vi "Main_FFT.vi"() -> ()   [LabVIEW 2026]
doc: "This template is for the Queued Message Handler design pattern.\n\nThe Event Handling Loop generates messages based on user interface actions.\n\nThe Message Handling Loop processes messages generated by the Event Handling Loop, or by other messages. The messages are string values, so new messages can be added easily to the Message Cases case structure in the Message Handling Loop. Each message cluster can also provide an optional value for Message Data, which is a variant that can be converted to whatever message-specific data is required."
uses:
  SubVIs/Controls/PCO_Config.ctl
  SubVIs/Controls/UI Data.ctl
  SubVIs/pco.labview/camera/Camera.lvclass
  SubVIs/Controls/TypeDef_FGV.ctl
  SubVIs/QMH/Message Queue/Enqueue Message (Single).vi
  SubVIs/QMH/Message Queue/Message Queue.lvlib
  SubVIs/QMH/User Event - Stop/User Event - Stop.lvlib
  SubVIs/pco.labview/pco.sdk/TimingControl/TimingControl.lvlib
panel:
  in  "# of frames":u16=100
  in  "SavePath":path=path "E:/exp_data/Seb"
  out "FFT":dbl[][](graph)
  out "Graphe d'intensité":u16[][](graph)
  in  "Binning for FFT":u16(ring)=8 items=["1x1"=1, "2x2"=2, "4x4"=4, "8x8"=8]
  in  "Stop live":bool
  in  "FFT?":bool=TRUE
  in  "Grab":bool
  in  "Live":bool
  in  "PCO_Config":T1={"Exposure time (s)"=0.01, "TriggerMode"=0, "ROI X0"=1, "ROI Y0"=1, "ROI X1"=2048, "ROI Y1"=2048, "Binning"=1} {"TriggerMode" items=["auto sequence", "software trigger", "external exposure start", "external exposure control"]}
  out "Current task":string="\"Exit\" button pressed"
  in  "Exit":bool
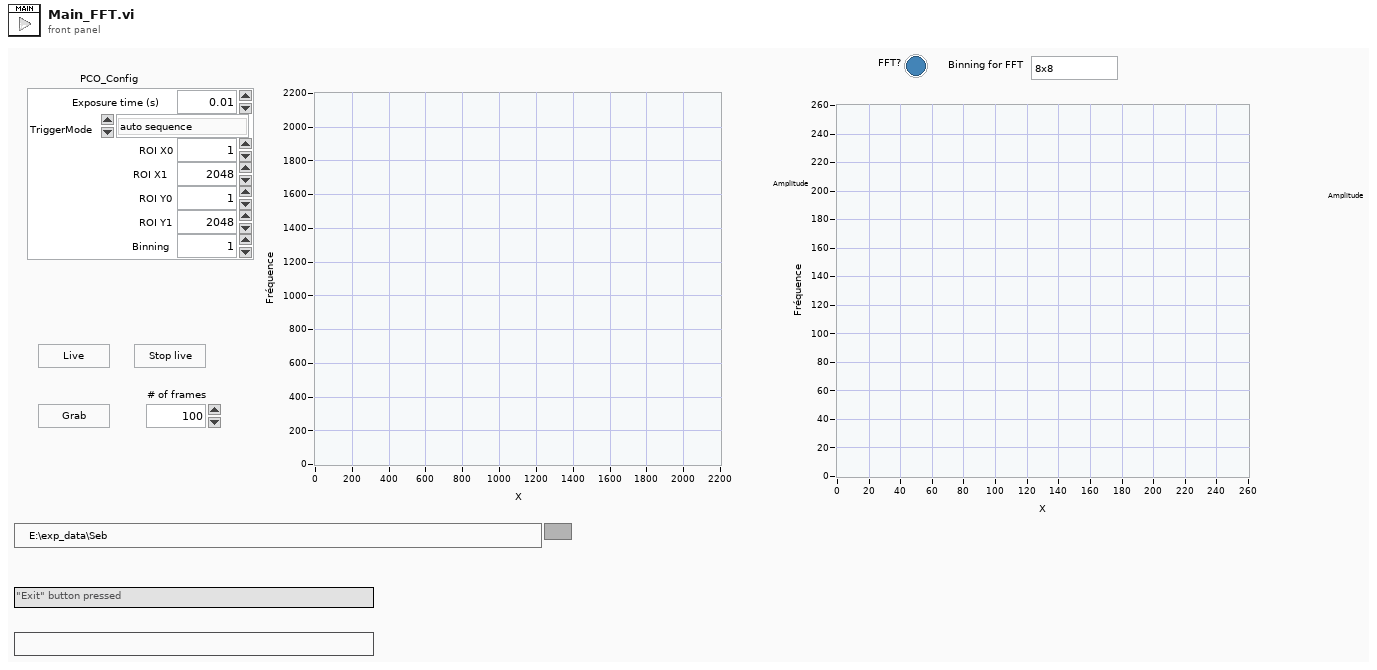
[diagram p1: front panel]
types:
  T1 = typedef "PCO_Config.ctl" = cluster{"Exposure time (s)":dbl, "TriggerMode":u16, "ROI X0":u16, "ROI Y0":u16, "ROI X1":u16, "ROI Y1":u16, "Binning":u8}
  T2 = typedef "UI Data.ctl" = cluster{"Data Display Ref":refnum<vi>, "Exit Button Ref":refnum<vi>, "Message":string}
  T3 = typedef "Message Queue.lvlib/All Message Queues.ctl" = cluster{"UI":refnum<queue>, "Camera loop":refnum<queue>, "Display loop":refnum<queue>}
  T4 = typedef "TypeDef_FGV.ctl" = enum16{"Initialize", "Write", "Read"}
  T5 = enum16{"auto sequence", "software trigger", "external exposure start", "external exposure control"}
  T6 = typedef "Camera.lvclass/binning.ctl" = cluster{"vert":u16, "horz":u16, "mode":u16}
  T7 = cluster{"exposure_time_s":dbl, "delay_time_s":dbl, "roi":cluster{"x0":u64, "y0":u64, "x1":u64, "y1":u64}, "timestamp_mode":u16, "pixelrate":u32, "conversion_factor":sgl, "trigger_mode":u16, "acquire_mode":u16, "acquire_sequence_number":u32, "metadata_mode":u16, "noisefilter_mode":u16, "pixel_format":u32, "binning":T6, "auto_exposure":cluster{"region":u16, "min_exposure_s":dbl, "max_exposure_s":dbl}}
  T8 = cluster{"wSignalNum":u16, "wEnabled":u16, "wType":u16, "wPolarity":u16, "wFilterSetting":u16, "wSelected":u16, "dwParameter":u32[], "dwSignalFunctionality":u32[]}
  T9 = cluster{"wVersion":u16, "dwIMAGE_COUNTER":u32, "dwIMAGE_TIME_US":u32, "lvTimestamp":timestamp, "bIMAGE_TIME_STATUS":u8, "wEXPOSURE_TIME_BASE":u16, "dwEXPOSURE_TIME":u32, "dwFRAMERATE_MILLIHZ":u32, "sSENSOR_TEMPERATURE":i16, "wIMAGE_SIZE_X":u16, "wIMAGE_SIZE_Y":u16, "bBINNING_X":u8, "bBINNING_Y":u8, "dwSENSOR_READOUT_FREQUENCY":u32, "wSENSOR_CONV_FACTOR":u16, "dwCAMERA_SERIAL_NO":u32, "wCAMERA_TYPE":u16, "bBIT_RESOLUTION":u8, "bSYNC_STATUS":u8, "wDARK_OFFSET":u16, "bTRIGGER_MODE":u8, "bDOUBLE_IMAGE_MODE":u8, "bCAMERA_SYNC_MODE":u8, "bIMAGE_TYPE":u8, "wCOLOR_PATTERN":u16, "wCAMERA_SUBTYPE":u16, "dwEVENT_NUMBER":u32, "wIMAGE_SIZE_X_Offset":u16, "wIMAGE_SIZE_Y_Offset":u16, "bREADOUT_MODE":u8}[]
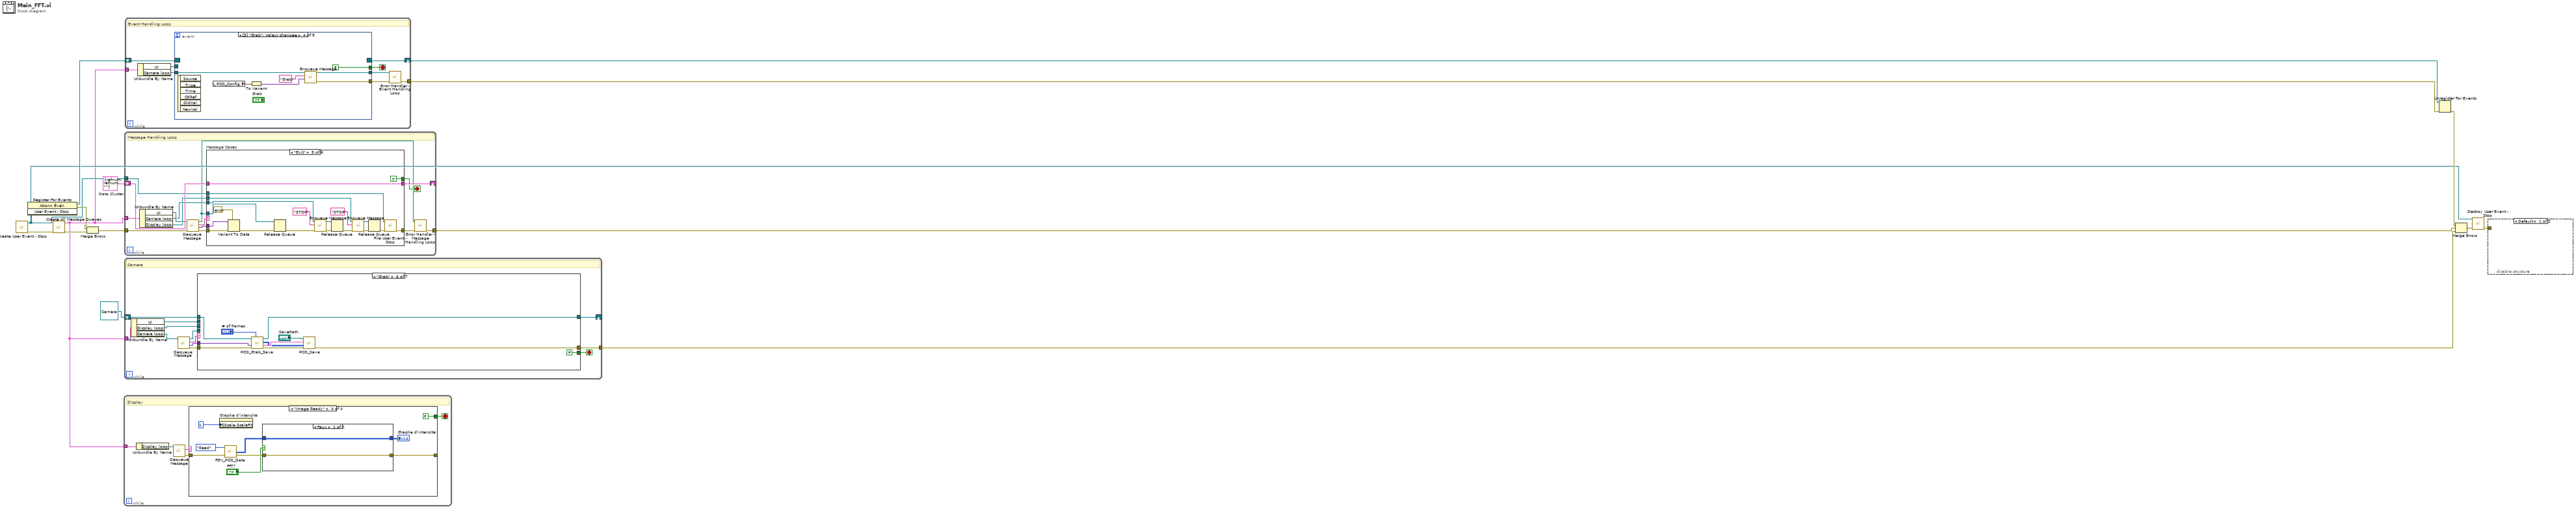
[diagram p0: block diagram]
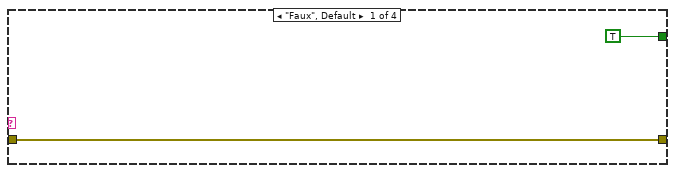
[diagram p2: hidden frame]
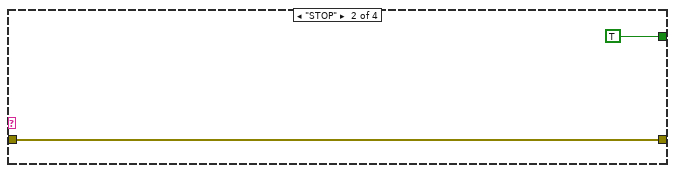
[diagram p3: hidden frame]
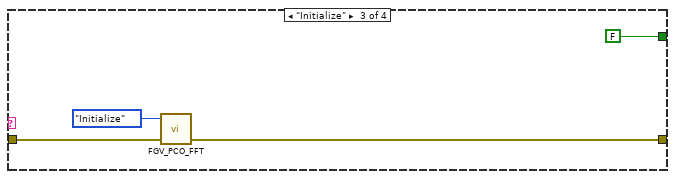
[diagram p4: hidden frame]
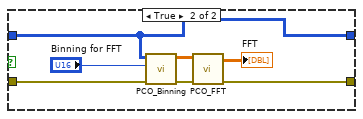
[diagram p5: hidden frame]
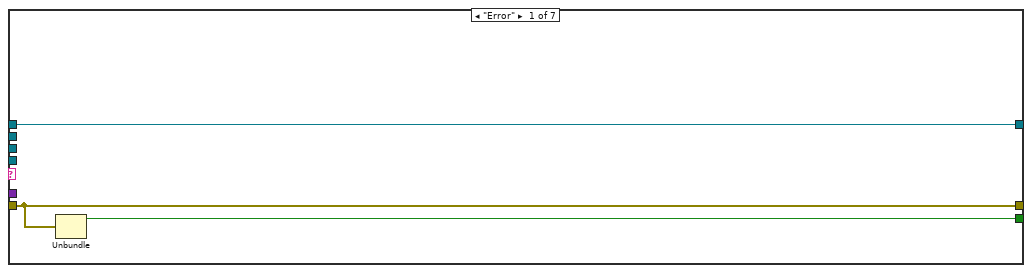
[diagram p6: hidden frame]
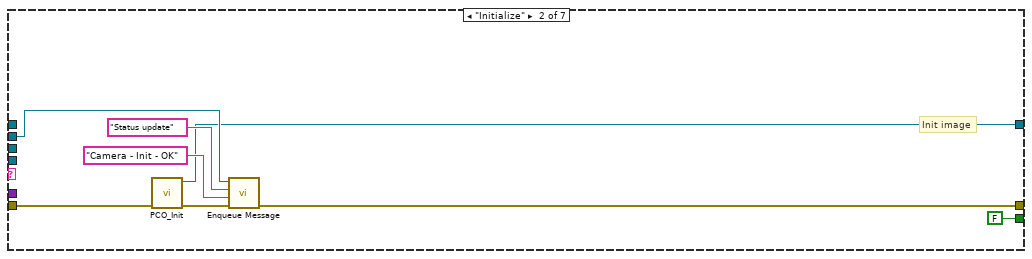
[diagram p7: hidden frame]
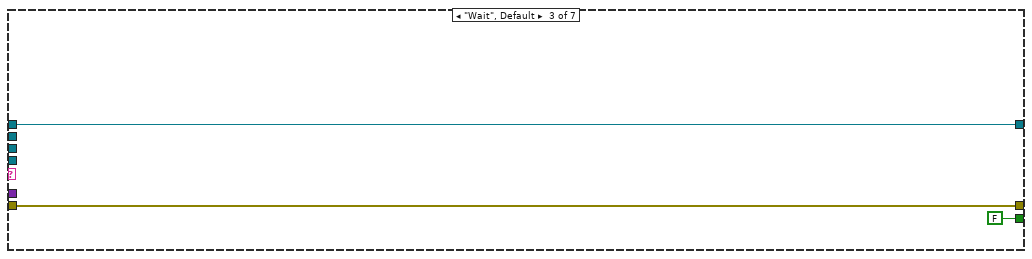
[diagram p8: hidden frame]
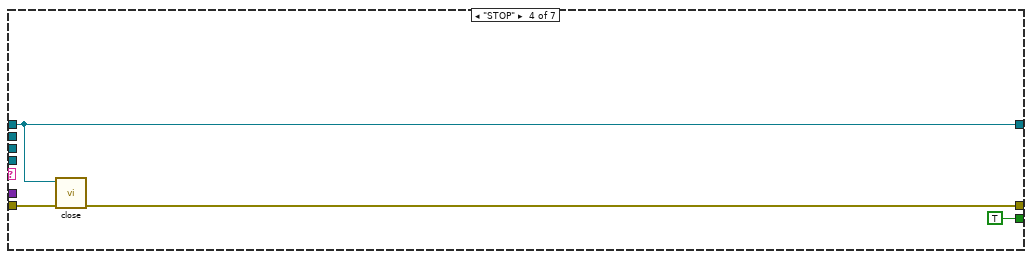
[diagram p9: hidden frame]
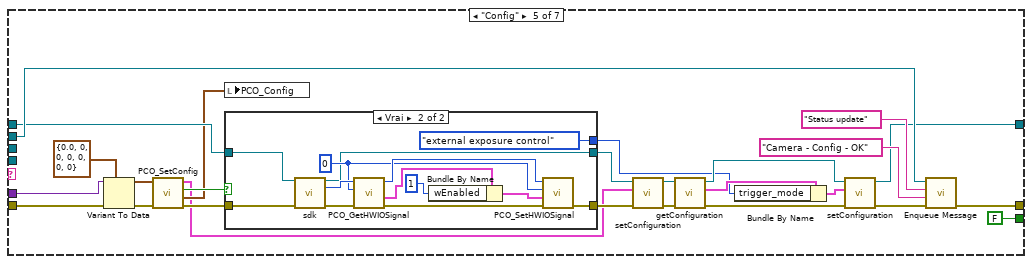
[diagram p10: hidden frame]
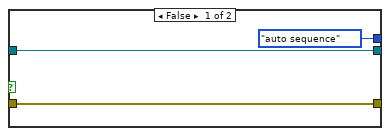
[diagram p11: hidden frame]
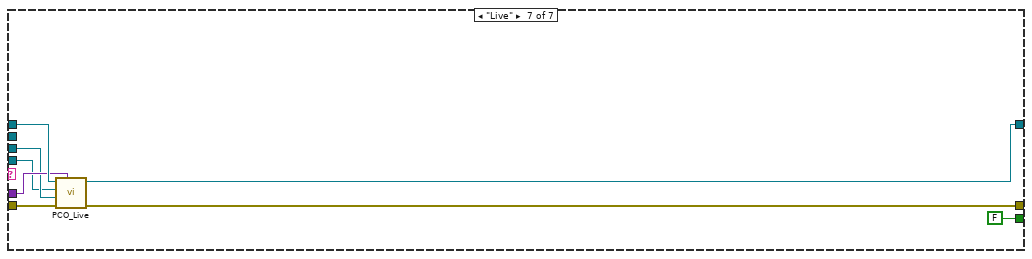
[diagram p12: hidden frame]
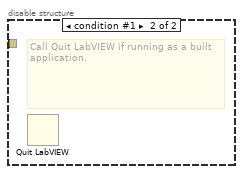
[diagram p13: hidden frame]
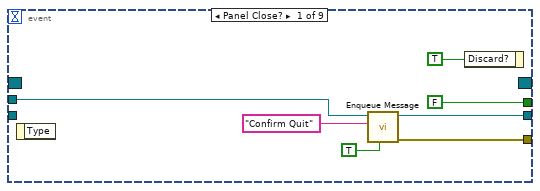
[diagram p14: hidden frame]
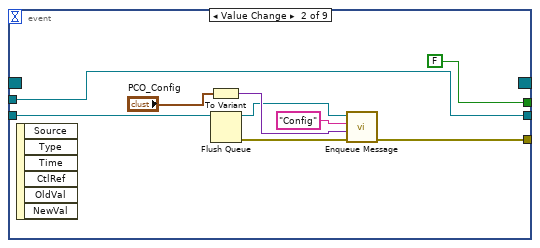
[diagram p15: hidden frame]
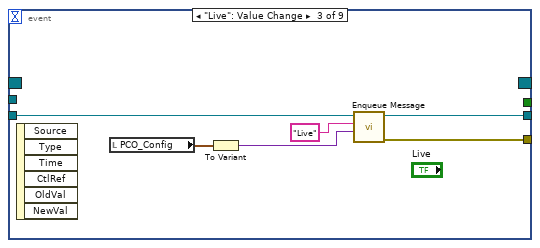
[diagram p16: hidden frame]
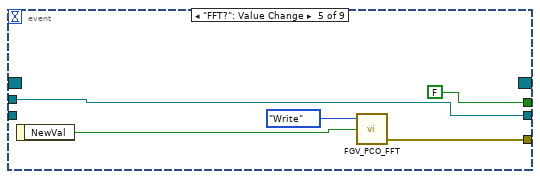
[diagram p17: hidden frame]
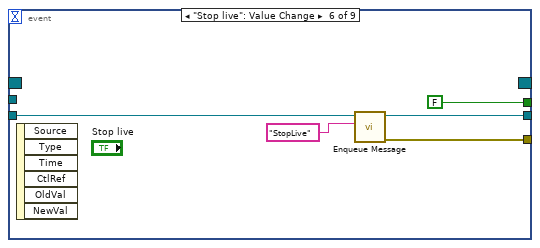
[diagram p18: hidden frame]
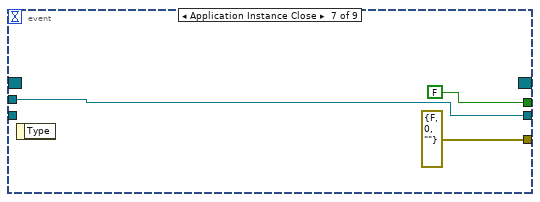
[diagram p19: hidden frame]
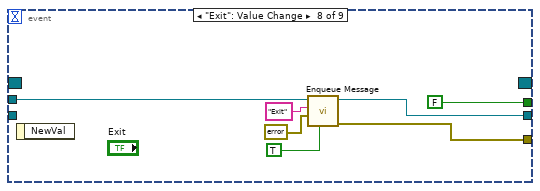
[diagram p20: hidden frame]
diagram:
  w4 = T2 {"Data Display Ref"=refnum, "Exit Button Ref"=refnum, "Message"=""}  # Data Cluster
  n1 = call "Create User Event - Stop.vi"() -> ("error out"=w14:errorcluster, "User Event - Stop"=w7:refnum<user-event>)  [unwired: 10 in]
  n2 = register-events(w7) -> (reference out=w8:refnum<event-registration>, error out=w5:errorcluster)  [unwired: 2 in]
  n3 = call "Create All Message Queues.vi"("error in (no error)"=w14) -> ("error out"=w16:errorcluster, "Message Queues out"=w2:T3)  [unwired: 9 in]
  n4 = Merge Errors(w5, w16) -> (w6:errorcluster)
  n5 = while {
    tunnel: w2 -> [w21]
    stop <- w17 stop-if-true
    # "Display"
    n6 = Unbundle By Name(w21) -> ("Display loop"=w20:refnum<queue>)
    n7 = call "Dequeue Message.vi"("Message Queue"=w20) -> ("error out"=w18:errorcluster, "Message"=w19:string)  [unwired: 7 in, 2 out]
    n8 = case shown="\"Image Ready\"" w19 {
      tunnel: w18 -> [w23 w24 w28 w37]
      tunnel: [w23 w24 w27 w31] -> _
      tunnel: [TRUE TRUE FALSE FALSE] -> w17
      frame "Faux", Default {
      }
      frame "STOP" {
      }
      frame "Initialize" {
        n9 = call "FGV_PCO_FFT.vi"("error in"=w28, "Action"=TypeDef_FGV."Initialize") -> ("error out"=w27:errorcluster)  [unwired: 2 in, 1 out]
      }
      frame "Image Ready" {
        n10 = property on="Graphe d'intensité" class="GraphInt (strict)"("ZScale.ScaleFit"=u8 1 ("Échelle des Z.Ajuster l'échelle")) -> ()  [unwired: 2 in, 2 out]
        n11 = call "FGV_PCO_Data.vi"("error in"=w37, "Action"=TypeDef_FGV."Read") -> ("error out"=w35:errorcluster, "Data"=w34:u16[][])  [unwired: 2 in]
        n12 = case shown="Faux" "FFT?" {
          tunnel: [w40 w41] -> w31
          tunnel: w35 -> [w40 w47]
          tunnel: w34 -> [w39 w44]
          tunnel: [w39 w44] -> w32
          frame False {
          }
          frame True {
            n13 = call "PCO_Binning.vi"("error in"=w47, "Binning"="Binning for FFT", "Data"=w44) -> ("error out"=w46:errorcluster, "Data bin"=w45:dbl[][])  [unwired: 7 in]
            n14 = call "PCO_FFT.vi"("error in (no error)"=w46, "Data"=w45) -> ("error out"=w41:errorcluster, "FFT"=→"FFT":dbl[][])  [unwired: 8 in]
          }
        }
        "Graphe d'intensité" <- w32
      }
    }
  }
  n15 = while {
    tunnel: [w55] -> w3
    tunnel: w2 -> [w54]
    shift-right: [w52] -> _
    shift-left: refnum<class "Camera.lvclass"> refnum ("Camera out") -> [w51]
    stop <- w56 stop-if-true
    # "Camera"
    n16 = Unbundle By Name(w54) -> ("UI"=w53:refnum<queue>, "Display loop"=w49:refnum<queue>, "Camera loop"=w48:refnum<queue>)
    n17 = call "Dequeue Message.vi"("Message Queue"=w48) -> ("error out"=w59:errorcluster, "Message Data"=w57:variant, "Message"=w58:string, "dup Message Queue"=w50:refnum<queue>)  [unwired: 7 in]
    n18 = case shown="\"Grab\"" w58 {
      tunnel: w59 -> [w62 w66 w73 w76 w102 w127 w136]
      tunnel: w57 -> [_ _ _ _ w101 w126 w135]
      tunnel: w53 -> [_ w70 _ _ w97 _ _]
      tunnel: [w61 FALSE ("status") FALSE ("status") TRUE FALSE ("status") FALSE ("status") FALSE ("status")] -> w56
      tunnel: [w62 w64 w73 w75 w96 w120 w133] -> w55
      tunnel: w50 -> [_ _ _ _ _ _ w131]
      tunnel: [w60 w65 w72 w74 w84 w130 w132] -> w52
      tunnel: w51 -> [w60 _ w72 w74 w92 w125 w137]
      tunnel: w49 -> [_ _ _ _ _ _ w134]
      frame "Error" {
        n19 = Unbundle(w62) -> ("status"=w61:bool)  [unwired: 2 out]
      }
      frame "Initialize" {
        # "Init image"
        n20 = call "PCO_Init.vi"("entrée d'erreur (pas d'erreur)"=w66) -> ("sortie d'erreur"=w63:errorcluster, "Camera en sortie"=w65:refnum<class "Camera.lvclass">)  [unwired: 9 in]
        n21 = call-poly "Enqueue Message.vi"("error in (no error)"=w63, "Message Data"="Camera - Init - OK", "Message"="Status update", "Message Queue"=w70) -> ("error out"=w64:errorcluster)  [unwired: 6 in, 1 out]
      }
      frame "Wait", Default {
      }
      frame "STOP" {
        n22 = call-dynamic "close.vi"("error in (no error)"=w76, "Camera in"=w74) -> ("error out"=w75:errorcluster)  [unwired: 9 in]
      }
      frame "Config" {
        n23 = Variant To Data(error in=w102, type=T1 {"Exposure time (s)"=0.0, "TriggerMode"=0, "ROI X0"=0, "ROI Y0"=0, "ROI X1"=0, "ROI Y1"=0, "Binning"=0} ("PCO_Config"), Variant=w101) -> (data=w99:T1, error out=w89:errorcluster)
        n24 = call "PCO_SetConfig.vi"("error in"=w89, "PCO_Config"=w99) -> ("error out"=w88:errorcluster, "PCO_Config 2"=w86:T1, "Trigger externe?"=w90:bool, "configuration"=w78:T7)  [unwired: 6 in]
        n25 = local write "PCO_Config"(w86) -> ()
        n26 = case shown="Vrai" w90 {
          tunnel: w88 -> [w106 w112]
          tunnel: [w106 w107] -> w93
          tunnel: w92 -> [w105 w110]
          tunnel: [w105 w109] -> w91
          tunnel: [T5."auto sequence" ("TriggerMode") T5."external exposure control" ("TriggerMode")] -> w79
          frame False {
          }
          frame True {
            w114 = u16 0 ("wSignalNum")
            n27 = call-dynamic "sdk.vi"("Camera in"=w110, "error in (no error)"=w112) -> ("Camera out"=w109:refnum<class "Camera.lvclass">, "sdk"=w115:u64, "error out"=w111:errorcluster)  [unwired: 11 in]
            n28 = call "PCO_GetHWIOSignal.vi"("error in (no error)"=w111, "wSignalNum"=w114, "ph"=w115) -> ("error out"=w117:errorcluster, "strSignal"=w119:T8, "ph out"=w116:u64)  [unwired: 5 in, 1 out]
            n29 = Bundle By Name(cluster=w119, "wEnabled"=u16 1) -> (w118:T8)
            n30 = call "PCO_SetHWIOSignal.vi"("error in (no error)"=w117, "strSignal"=w118, "wSignalNum"=w114, "ph"=w116) -> ("error out"=w107:errorcluster)  [unwired: 5 in, 2 out]
          }
        }
        n31 = call-dynamic "setConfiguration.vi"("error in (no error)"=w93, "configuration"=w78, "Camera in"=w91) -> ("error out"=w87:errorcluster, "Camera out"=w94:refnum<class "Camera.lvclass">)  [unwired: 7 in]
        n32 = call-dynamic "getConfiguration.vi"("error in (no error)"=w87, "Camera in"=w94) -> ("error out"=w83:errorcluster, "configuration"=w81:T7, "Camera out"=w85:refnum<class "Camera.lvclass">)  [unwired: 7 in]
        n33 = Bundle By Name(cluster=w81, "trigger_mode"=w79) -> (w80:T7)
        n34 = call-dynamic "setConfiguration.vi"("error in (no error)"=w83, "configuration"=w80, "Camera in"=w85) -> ("error out"=w82:errorcluster, "Camera out"=w84:refnum<class "Camera.lvclass">)  [unwired: 7 in]
        n35 = call-poly "Enqueue Message.vi"("error in (no error)"=w82, "Message Data"="Camera - Config - OK", "Message"="Status update", "Message Queue"=w97) -> ("error out"=w96:errorcluster)  [unwired: 6 in, 1 out]
      }
      frame "Grab" {
        n36 = call "PCO_Grab_Save.vi"("# of frames"="# of frames", "entrée d'erreur (pas d'erreur)"=w127, "Message Data"=w126, "Camera en entrée"=w125) -> ("sortie d'erreur"=w123:errorcluster, "meta_data_list"=w122:T9, "Raw data (U16)"=w121:u16[][][], "Camera en sortie"=w130:refnum<class "Camera.lvclass">)  [unwired: 4 in]
        n37 = call "PCO_Save.vi"("entrée d'erreur (pas d'erreur)"=w123, "raw_image_list (U16)"=w121, "meta_data_list"=w122, "SavePath"="SavePath") -> ("sortie d'erreur"=w120:errorcluster)  [unwired: 7 in]
      }
      frame "Live" {
        n38 = call "PCO_Live.vi"("Message Data"=w135, "entrée d'erreur (pas d'erreur)"=w136, "Display loop"=w134, "dup Message Queue"=w131, "Camera en entrée"=w137) -> ("sortie d'erreur"=w133:errorcluster, "Camera en sortie"=w132:refnum<class "Camera.lvclass">)  [unwired: 5 in]
      }
    }
  }
  n39 = while {
    shift-right: [w152] -> _
    shift-left: w4 -> [w153]
    tunnel: w7 -> [w150]
    tunnel: w6 -> [w149]
    tunnel: [w144] -> w15
    tunnel: w2 -> [w142]
    stop <- w151 stop-if-true
    # "Message Handling Loop"
    n40 = Unbundle By Name(w142) -> ("UI"=w141:refnum<queue>, "Camera loop"=w140:refnum<queue>, "Display loop"=w139:refnum<queue>)
    n41 = call "Dequeue Message.vi"("error in (no error)"=w149, "Message Queue"=w141) -> ("error out"=w148:errorcluster, "Message Data"=w146:variant, "Message"=w147:string, "dup Message Queue"=w145:refnum<queue>)  [unwired: 6 in]
    n42 = case "Message Cases" shown="\"Exit\"" w147 {
      tunnel: w145 -> [w156 _ _ w178 w192 _]
      tunnel: w148 -> [w161 w167 w174 w180 w193 w201]
      tunnel: [w162 w164 w169 w175 w188 w201] -> w143
      tunnel: w153 -> [w160 w168 w173 w179 w200 w202]
      tunnel: [w159 w168 w173 w179 w200 w202] -> w152
      tunnel: [_ _ _ _ TRUE _] -> w151
      tunnel: w146 -> [_ w166 w172 _ w196 _]
      tunnel: w150 -> [_ _ _ _ w198 _]
      tunnel: w140 -> [_ _ _ _ w191 _]
      tunnel: w139 -> [_ _ _ _ w181 _]
      frame "Initialize" {
        w154 = "Initial Message" ("Initial Message")
        n43 = control-ref of="Current task"() -> (w155:refnum<vi>)
        n44 = control-ref of="Exit"() -> (w158:refnum<vi>)
        n45 = Bundle By Name(cluster=w160, "Data Display Ref"=w155, "Exit Button Ref"=w158, "Message"=w154) -> (w159:T2)
        n46 = call-poly "Enqueue Message.vi"("error in (no error)"=w161, "Message Data"=w154, "Message"="Update Display", "Message Queue"=w156) -> ("error out"=w162:errorcluster)  [unwired: 6 in, 1 out]
      }
      frame "Update Display" {
        n47 = Variant To Data(error in=w167, type="", Variant=w166) -> (data=→"Current task":string, error out=w164:errorcluster)
      }
      frame "Error" {
        n48 = Variant To Data(error in=w174, type=errorcluster {"status"=FALSE, "code"=0, "source"=""} ("error constant"), Variant=w172) -> (data=w170:errorcluster, error out=w169:errorcluster)
        n49 = call <vilib>:"Simple Error Handler.vi"("error in (no error)"=w170) -> ()  [unwired: 4 in, 5 out]
      }
      frame "Confirm Quit" {
        n50 = call-poly "Enqueue Message.vi"("Priority Message? (F)"=TRUE, "error in (no error)"=w180, "Message"="Exit", "Message Queue"=w178) -> ("error out"=w175:errorcluster)  [unwired: 6 in, 1 out]
      }
      frame "Exit" {
        n51 = Variant To Data(error in=w193, type=errorcluster {"status"=FALSE, "code"=0, "source"=""} ("error constant"), Variant=w196) -> (error out=w189:errorcluster)  [unwired: 1 out]
        n52 = Release Queue(queue=w192, error in (no error)=w189) -> (error out=w187:errorcluster)  [unwired: 1 in, 2 out]
        n53 = call-poly "Enqueue Message.vi"("error in (no error)"=w187, "Message"="STOP", "Message Queue"=w191) -> ("error out"=w195:errorcluster, "dup Message Queue"=w194:refnum<queue>)  [unwired: 7 in]
        n54 = Release Queue(queue=w194, error in (no error)=w195) -> (error out=w183:errorcluster)  [unwired: 1 in, 2 out]
        n55 = call-poly "Enqueue Message.vi"("error in (no error)"=w183, "Message"="STOP", "Message Queue"=w181) -> ("error out"=w184:errorcluster, "dup Message Queue"=w185:refnum<queue>)  [unwired: 7 in]
        n56 = Release Queue(queue=w185, error in (no error)=w184) -> (error out=w182:errorcluster)  [unwired: 1 in, 2 out]
        n57 = call "Fire User Event - Stop.vi"("error in (no error)"=w182, "User Event - Stop"=w198) -> ("error out"=w188:errorcluster)  [unwired: 9 in]
      }
      frame Default {
      }
    }
    n58 = call "Error Handler - Message Handling Loop.vi"("error in (no error)"=w143, "Message Queue"=w145) -> ("dup error in"=w144:errorcluster)  [unwired: 8 in, 1 out]
  }
  n59 = while {
    shift-right: [w210] -> w11
    shift-left: w8 -> [w211]
    tunnel: [w206] -> w9
    tunnel: w2 -> [w203]
    stop <- w208 stop-if-true
    # "Event Handling Loop"
    n60 = Unbundle By Name(w203) -> ("UI"=w205:refnum<queue>, "Camera loop"=w204:refnum<queue>)
    n61 = event shown="[3] \"Grab\": Valeur changée" {
      selector: w211 -> [_ _ _ _ _ _ _ _ _]
      dyn-events: [_ _ _ _ _ _ _ _ _] -> w210
      timeout: _ -> [_ _ _ _ _ _ _ _ _]
      tunnel: [FALSE ("Discard?") FALSE ("Discard?") _ FALSE ("Discard?") FALSE ("Discard?") FALSE ("Discard?") FALSE ("Discard?") FALSE ("Discard?") TRUE ("Discard?")] -> w208
      tunnel: w205 -> [w217 w227 _ _ w245 _ w253 w260 w264]
      tunnel: [w216 w223 w230 w237 w243 w248 errorcluster {"status"=FALSE, "code"=0, "source"=""} ("error out") w254 errorcluster {"status"=FALSE, "code"=0, "source"=""} ("error out")] -> w209
      tunnel: [w215 w227 w229 w238 w245 w247 w253 w259 w264] -> w207
      tunnel: w204 -> [_ w221 w228 w239 _ w249 _ _ _]
      event Panel Close? {
        n62 = event-data() -> ()  [unwired: 1 in, 1 out]
        n63 = call-poly "Enqueue Message.vi"("Priority Message? (F)"=TRUE, "Message"="Confirm Quit", "Message Queue"=w217) -> ("error out"=w216:errorcluster, "dup Message Queue"=w215:refnum<queue>)  [unwired: 7 in]
        n64 = event-data("Discard?"=TRUE) -> ()  [unwired: 1 in, 1 out]
      }
      event Value Change {
        n65 = event-data() -> ()  [unwired: 1 in, 6 out]
        n66 = To Variant(anything="PCO_Config") -> (Variant=w224:variant)
        n67 = Flush Queue(queue=w221) -> (queue out=w219:refnum<queue>, error out=w220:errorcluster)  [unwired: 1 in, 1 out]
        n68 = call-poly "Enqueue Message.vi"("error in (no error)"=w220, "Message Data"=w224, "Message"="Config", "Message Queue"=w219) -> ("error out"=w223:errorcluster)  [unwired: 6 in, 1 out]
      }
      event "Live": Value Change {
        n69 = event-data() -> ()  [unwired: 1 in, 6 out]
        n70 = local read "PCO_Config"() -> (w233:T1)
        n71 = To Variant(anything=w233) -> (Variant=w232:variant)
        n72 = call-poly "Enqueue Message.vi"("Message Data"=w232, "Message"="Live", "Message Queue"=w228) -> ("error out"=w230:errorcluster, "dup Message Queue"=w229:refnum<queue>)  [unwired: 7 in]
      }
      event "Grab": Value Change {
        n73 = event-data() -> ()  [unwired: 1 in, 6 out]
        n74 = local read "PCO_Config"() -> (w235:T1)
        n75 = To Variant(anything=w235) -> (Variant=w234:variant)
        n76 = call-poly "Enqueue Message.vi"("Message Data"=w234, "Message"="Grab", "Message Queue"=w239) -> ("error out"=w237:errorcluster, "dup Message Queue"=w238:refnum<queue>)  [unwired: 7 in]
      }
      event "FFT?": Value Change {
        n77 = event-data() -> ("NewVal"=w241:bool)  [unwired: 1 in]
        n78 = call "FGV_PCO_FFT.vi"("FFT?"=w241, "Action"=TypeDef_FGV."Write") -> ("error out"=w243:errorcluster)  [unwired: 2 in, 1 out]
      }
      event "Stop live": Value Change {
        n79 = event-data() -> ()  [unwired: 1 in, 6 out]
        n80 = call-poly "Enqueue Message.vi"("Message"="StopLive", "Message Queue"=w249) -> ("error out"=w248:errorcluster, "dup Message Queue"=w247:refnum<queue>)  [unwired: 8 in]
      }
      event Application Instance Close {
        n81 = event-data() -> ()  [unwired: 1 in, 1 out]
      }
      event "Exit": Value Change {
        n82 = event-data() -> ()  [unwired: 1 in, 1 out]
        n83 = call-poly "Enqueue Message.vi"("Priority Message? (F)"=TRUE, "Message Data"=errorcluster {"status"=FALSE, "code"=0, "source"=""} ("error constant"), "Message"="Exit", "Message Queue"=w260) -> ("error out"=w254:errorcluster, "dup Message Queue"=w259:refnum<queue>)  [unwired: 6 in]
      }
      event User Event {
        n84 = event-data() -> ()  [unwired: 1 in, 1 out]
        n85 = local write "Current task"("\"Exit\" button pressed" ("VI Stopped")) -> ()
      }
    }
    n86 = call "Error Handler - Event Handling Loop.vi"("error in (no error)"=w209, "Message Queue"=w207) -> ("dup error in"=w206:errorcluster)  [unwired: 8 in, 1 out]
  }
  n87 = Unregister For Events(event registration refnum=w11, error in=w9) -> (error out=w12:errorcluster)
  n88 = Merge Errors(w12, w15, w3) -> (w13:errorcluster)
  n89 = call "Destroy User Event - Stop.vi"("error in (no error)"=w13, "User Event - Stop"=w7) -> ("error out"=w10:errorcluster)  [unwired: 9 in]
  n90 = disable-structure shown="Default" {
    disable-tunnel: w10 -> [_ _]
    frame condition #0 (active) {
    }
    frame condition #1 {
      # "Call Quit LabVIEW if running as a built application."
      n91 = Quit LabVIEW() -> ()  [unwired: 1 in]
    }
  }
